vi "Call And Receive.vi"(6 "timeout in ms (-1)":i32=-1, 8 "error in (no error)":errorcluster, 9 "Parameter":variant, 10 "Function":string, 11 "input in":refnum<class "Input.lvclass">) -> (0 "error out":errorcluster, 1 "timeout":bool, 2 "Data":variant, 3 "input out":refnum<class "Input.lvclass">)   [LabVIEW 2015, in "Input.lvclass"]
uses:
  Input.lvclass
  Result/result_from_call/result_from_call.lvclass
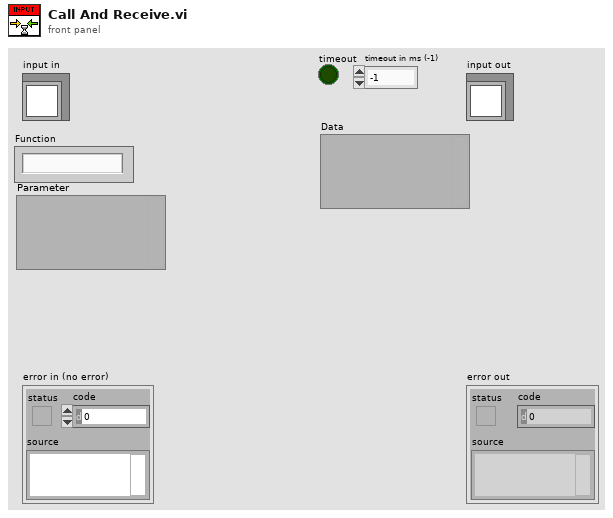
[diagram p1: front panel]
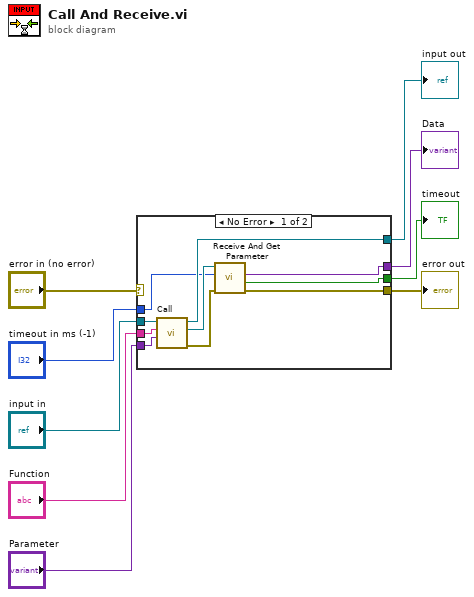
[diagram p0: block diagram]
diagram:
  n1 = case shown="No Error" "error in (no error)" {
    selector: "error in (no error)" -> [_ w21]
    tunnel: [w14 w21] -> w8
    tunnel: [w11 w20] -> w6
    tunnel: "input in" -> [w15 w20]
    tunnel: "Parameter" -> [w16 _]
    tunnel: "Function" -> [w17 _]
    tunnel: [w13 _] -> w3
    tunnel: [w12 _] -> w2
    tunnel: "timeout in ms (-1)" -> [w10 _]
    frame No Error {
      n2 = call "Call.vi"("Parameter"=w16, "Function"=w17, "input in"=w15) -> ("error out"=w18:errorcluster, "result"=w19:refnum<class "result_from_call.lvclass">, "input out"=w11:refnum<class "Input.lvclass">)  [unwired: 6 in]
      n3 = call "Receive And Get Parameter.vi"("error in (no error)"=w18, "timeout in ms (-1)"=w10, "result_from_call in"=w19) -> ("error out"=w14:errorcluster, "timeout"=w13:bool, "Data"=w12:variant)  [unwired: 5 in, 1 out]
    }
    frame Error {
    }
  }
  "error out" <- w8
  "input out" <- w6
  "Data" <- w2
  "timeout" <- w3
